vi "Get Acquire Settings.vi"(8 "error in (no error)":errorcluster, 10 "Time":T1 {"Time/Div" min=0.0 max=16.0 step=1.0 scale=0.0..12.0}) -> (0 "error out":errorcluster, 2 "# Elements to Read":u32, 3 "Acquire Rate":dbl)   [LabVIEW 2021]
uses:
  Controls/Time Selector.ctl
  Controls/Time Knob.ctl
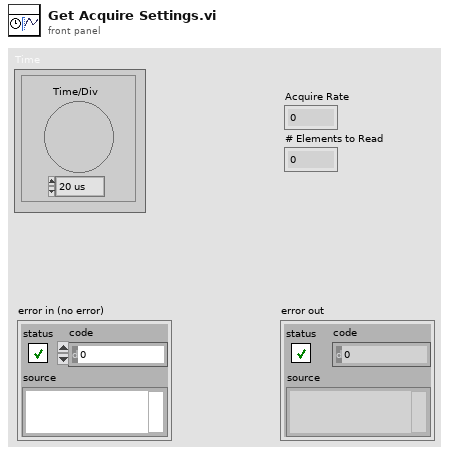
[diagram p1: front panel]
types:
  T1 = typedef "Time Selector.ctl" = cluster{"Time/Div":T2}
  T2 = typedef "Time Knob.ctl" = dbl
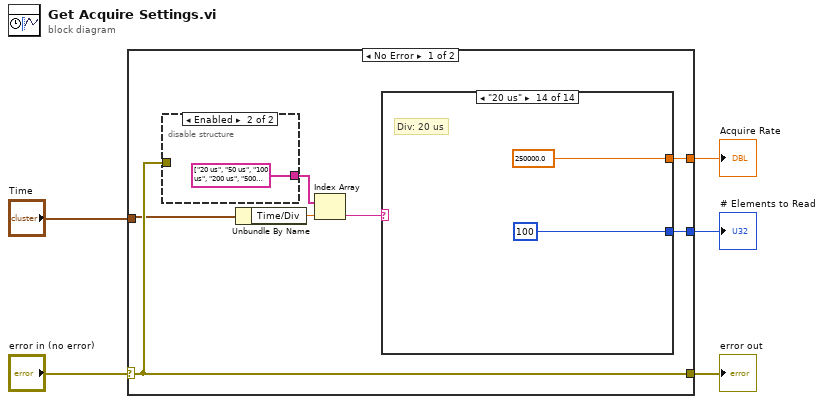
[diagram p0: block diagram]
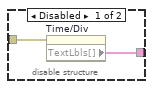
[diagram p2: hidden frame]
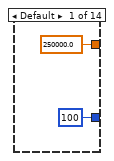
[diagram p3: hidden frame]
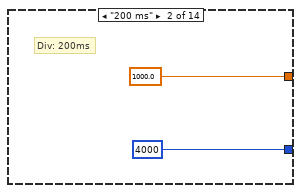
[diagram p4: hidden frame]
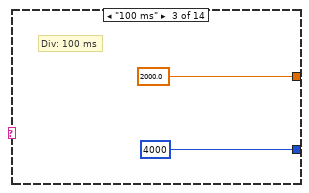
[diagram p5: hidden frame]
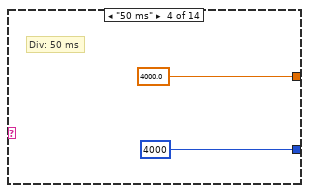
[diagram p6: hidden frame]
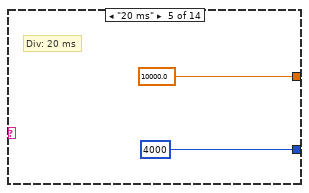
[diagram p7: hidden frame]
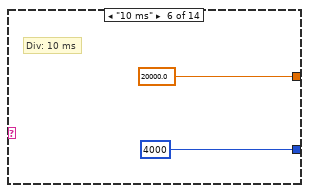
[diagram p8: hidden frame]
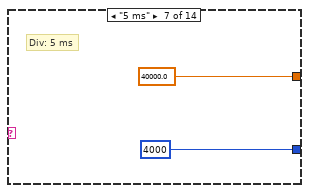
[diagram p9: hidden frame]
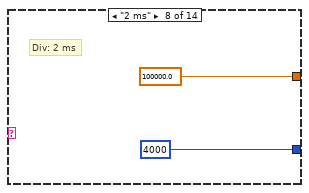
[diagram p10: hidden frame]
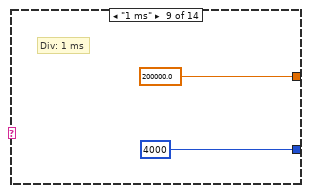
[diagram p11: hidden frame]
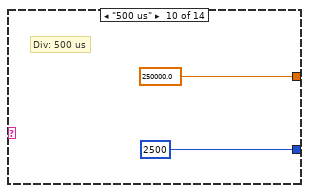
[diagram p12: hidden frame]
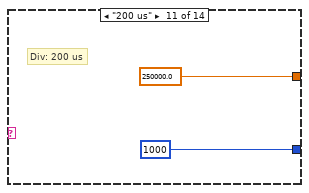
[diagram p13: hidden frame]
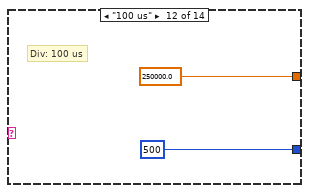
[diagram p14: hidden frame]
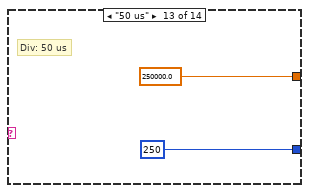
[diagram p15: hidden frame]
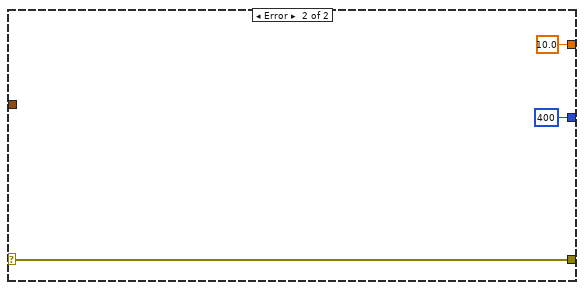
[diagram p16: hidden frame]
diagram:
  n1 = case shown="No Error" "error in (no error)" {
    selector: "error in (no error)" -> [w8 w44]
    tunnel: "Time" -> [w7 _]
    tunnel: [w12 10.0] -> w4
    tunnel: [w11 u32 400] -> w3
    tunnel: [w8 w44] -> w1
    frame No Error {
      n2 = disable-structure shown="Enabled" {
        disable-tunnel: [w14 string[] ["20 us", "50 us", "100 us", "200 us", "500 us", "1 ms", "2 ms", "5 ms", "10 ms", "20 ms", "50 ms", "100 ms", "200 ms"] ("Text Labels[]")] -> w10
        disable-tunnel: w8 -> [w13 _]
        frame Disabled {
          n3 = property on="Time/Div" class="Knob (strict)"(error in=w13) -> ("TextLbls[]"=w14:string[])  [unwired: 1 in, 2 out]
        }
        frame Enabled {
        }
      }
      n4 = Unbundle By Name(w7) -> ("Time/Div"=w6:T2)
      n5 = Index Array(array=w10, index=w6) -> (element=w9:string)
      n6 = case shown="\"20 us\"" w9 {
        tunnel: [250000.0 1000.0 2000.0 4000.0 10000.0 20000.0 40000.0 100000.0 200000.0 250000.0 250000.0 250000.0 250000.0 250000.0] -> w12
        tunnel: [u32 100 u32 4000 u32 4000 u32 4000 u32 4000 u32 4000 u32 4000 u32 4000 u32 4000 u32 2500 u32 1000 u32 500 u32 250 u32 100] -> w11
        frame Default {
        }
        frame "200 ms" {
          # "Div: 200ms"
        }
        frame "100 ms" {
          # "Div: 100 ms"
        }
        frame "50 ms" {
          # "Div: 50 ms"
        }
        frame "20 ms" {
          # "Div: 20 ms"
        }
        frame "10 ms" {
          # "Div: 10 ms"
        }
        frame "5 ms" {
          # "Div: 5 ms"
        }
        frame "2 ms" {
          # "Div: 2 ms"
        }
        frame "1 ms" {
          # "Div: 1 ms"
        }
        frame "500 us" {
          # "Div: 500 us"
        }
        frame "200 us" {
          # "Div: 200 us"
        }
        frame "100 us" {
          # "Div: 100 us"
        }
        frame "50 us" {
          # "Div: 50 us"
        }
        frame "20 us" {
          # "Div: 20 us"
        }
      }
    }
    frame Error {
    }
  }
  "Acquire Rate" <- w4
  "# Elements to Read" <- w3
  "error out" <- w1
